vi "FPGA Main.vi"() -> ()   [LabVIEW 2009]
uses:
  <vilib>/rvi/DataTransferAndStorage/Container/XNode/niFpgaContainer.xnode
  <vilib>/rvi/FIFO/Fifo_Resource/nirvififoUniquifyingName.vi
panel:
  in  "stop bits (10: 1 bit)":u16(ring)=10 items=["1.0"=10, "1.5"=15, "2.0"=20]
  in  "parity (0:none)":enum16{"None", "Odd", "Even", "Mark", "Space"}(ring)
  in  "data bits (8)":i32=8 min=5 max=8 step=1
  in  "stop":bool
  in  "Write: Char":u8
  in  "Write: Data Written":bool
  in  "baud rate (9600)":u32=9600
  in  "Invert Polarity?":bool
  out "Read: Char":u8
  out "Read: New Data":bool
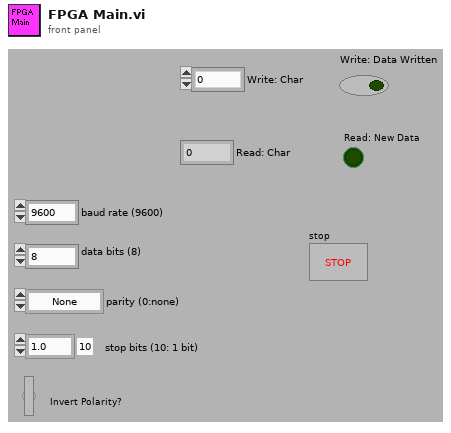
[diagram p1: front panel]
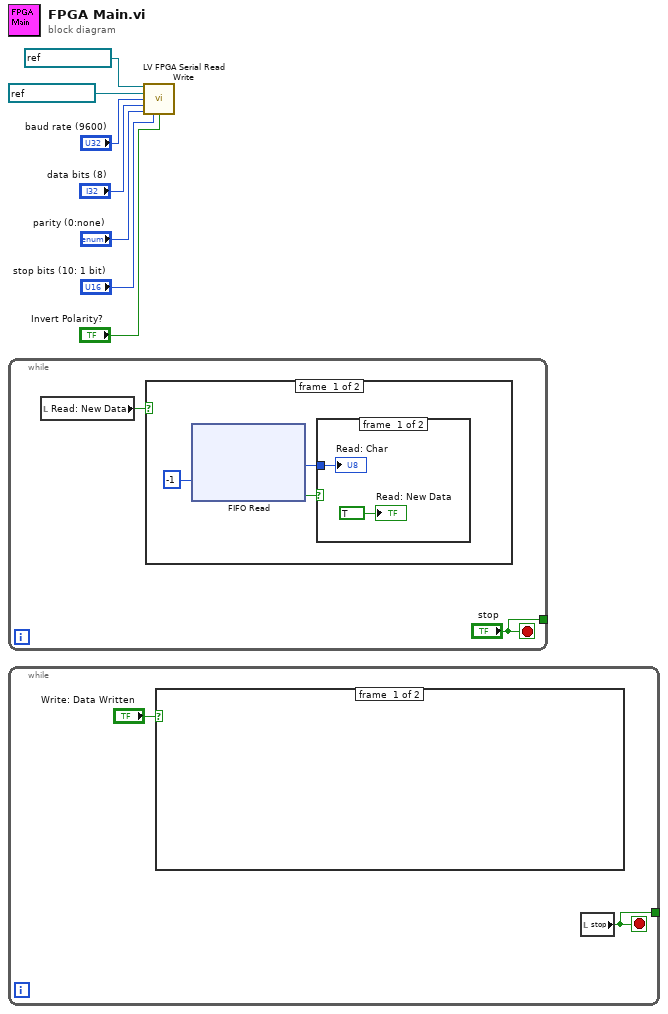
[diagram p0: block diagram]
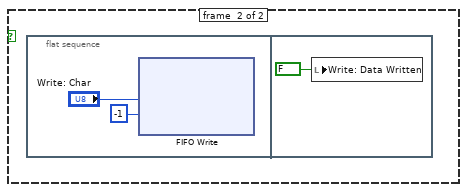
[diagram p4: hidden frame]
diagram:
  n1 = while {
    tunnel: ["stop"] -> _
    stop <- "stop" stop-if-true
    n2 = local read "Read: New Data"() -> (w9:bool)
    n3 = case shown="False" w9 {
      frame #0 {
        n4 = xnode ("FIFO Read")("Timeout"=-1) -> ("Element"=w10:u8, "Timed Out?"=w11:bool)  [unwired: 1 in, 1 out]
        n5 = case shown="False" w11 {
          tunnel: w10 -> [w62 _]
          frame #0 {
            "Read: Char" <- w62
            "Read: New Data" <- TRUE ("Read: New Data")
          }
          frame #1 {
          }
        }
      }
      frame #1 {
      }
    }
  }
  n6 = while {
    tunnel: [w63] -> _
    stop <- w63 stop-if-true
    n7 = case shown="True" "Write: Data Written" {
      frame #0 {
      }
      frame #1 {
        n8 = flat-sequence {
          frame #0 {
            n9 = xnode ("FIFO Write")("Element"="Write: Char", "Timeout"=-1) -> ()  [unwired: 1 in, 2 out]
          }
          frame #1 {
            n10 = local write "Write: Data Written"(FALSE ("Write: Data Written")) -> ()
          }
        }
      }
    }
    n11 = local read "stop"() -> (w63:bool)
  }
  n12 = call "LV FPGA Serial Read Write.vi"("Transmit"=refnum<k21> "Port4/DIO7", "Receive"=refnum<k21> "Port4/DIO8", "baud rate (9600)"="baud rate (9600)", "data bits (8)"="data bits (8)", "parity (0:none)"="parity (0:none)", "stop bits (10: 1 bit)"="stop bits (10: 1 bit)", "Invert Polarity?"="Invert Polarity?") -> ()  [unwired: 9 out]
